vi "Test Initiate.vi"(0 "Template Rx Test in":refnum<class "niDTS WLAN Rx Test.lvclass">, 11 "error in (no error)":errorcluster) -> (4 "Template Rx Test out":refnum<class "niDTS WLAN Rx Test.lvclass">, 15 "error out":errorcluster)   [LabVIEW 2015, in "niDTS WLAN.lvlib" / "niDTS WLAN Rx Test.lvclass"]
uses:
  niDTS WLAN Rx Test.lvclass
  niDTS WLAN Rx Test.lvclass/niDTS WLAN Rx Test.ctl
  Instrument/INSTR RX/niDTS WLAN INSTR RX.lvclass
  Framework/Dut/Objects/BASE_class/niDTS Dut.lvclass
  Dut/Objects/BASE_class/niDTS WLAN Dut.lvclass
  niDTS WLAN.lvlib
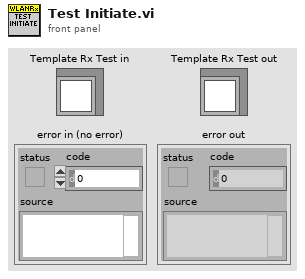
[diagram p1: front panel]
types:
  T1 = typedef "niDTS Framework.lvlib/niDTS Dut INC Handle.ctl" = refnum<data-value>
  T2 = typedef "niDTS WLAN.lvlib/niDTS WLAN Dut INC Handle.ctl" = refnum<data-value>
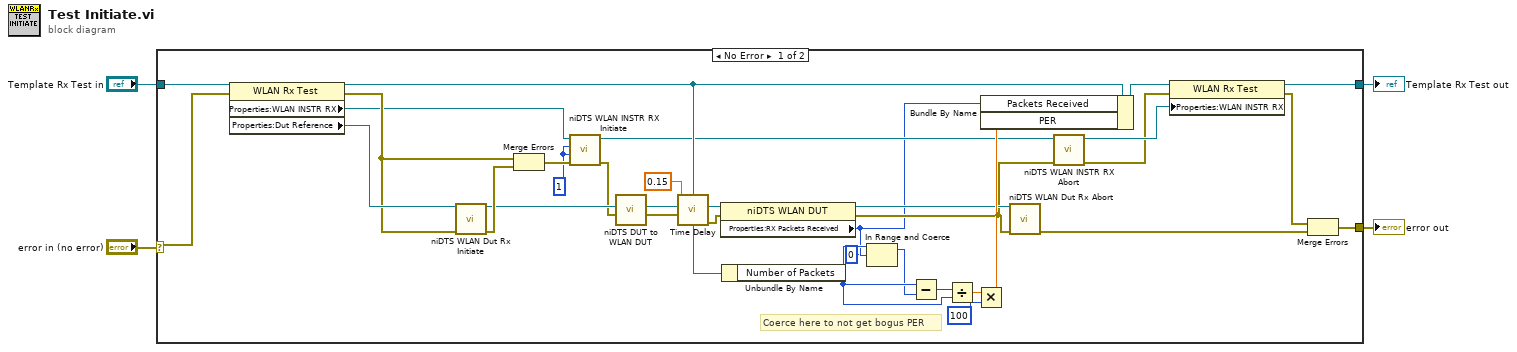
[diagram p0: block diagram]
diagram:
  n1 = case shown="No Error" "error in (no error)" {
    selector: "error in (no error)" -> [w37 w39]
    tunnel: [w12 w39] -> w3
    tunnel: [w11 w38] -> w1
    tunnel: "Template Rx Test in" -> [w36 w38]
    frame No Error {
      w27 = 1 ("Driver Instance")
      # "Coerce here to not get bogus PER"
      n2 = property class="WLAN Rx Test"(reference=w36, error in=w37) -> (reference out=w29:refnum<class "niDTS WLAN Rx Test.lvclass">, error out=w26:errorcluster, "Properties:WLAN INSTR RX"=w19:refnum<class "niDTS WLAN INSTR RX.lvclass">, "Properties:Dut Reference"=w35:T1)
      n3 = call "niDTS WLAN Dut Rx Initiate.vi"("Dut Handle in"=w35, "error in (no error)"=w26) -> ("Dut Handle out"=w23:T1, "error out"=w25:errorcluster)  [unwired: 12 in]
      n4 = Merge Errors(w26, w25) -> (w28:errorcluster)
      n5 = call-dynamic "niDTS WLAN INSTR RX Initiate.vi"("error in (no error)"=w28, "Result Instance"=w27, "Driver Instance"=w27, "niDTS WLAN INSTR RX in"=w19) -> ("error out"=w22:errorcluster, "niDTS WLAN INSTR RX out"=w20:refnum<class "niDTS WLAN INSTR RX.lvclass">)  [unwired: 6 in]
      n6 = call "niDTS DUT to WLAN DUT.vi"("error in"=w22, "Dut Handle"=w23) -> ("error out"=w18:errorcluster, "WLAN Dut Handle"=w21:T2)  [unwired: 8 in]
      n7 = call "Time Delay"("error in (no error)"=w18, "Delay Time (s)"=0.15) -> ("error out"=w17:errorcluster)  [unwired: 9 in]
      n8 = property class="niDTS WLAN DUT"(reference=w21, error in=w17) -> (reference out=w30:T2, error out=w9:errorcluster, "Properties:RX Packets Received"=w7:u32)
      n9 = Unbundle By Name(w29) -> ("Number of Packets"=w8:i32)
      n10 = In Range and Coerce(upper limit=w8, x=w7, lower limit=u32 0) -> (coerced(x)=w5:u32)  [unwired: 1 out]
      n11 = Subtract(x=w8, y=w5) -> (x-y=w34:u32)
      n12 = Divide(x=w34, y=w8) -> (x/y=w33:dbl)
      n13 = Multiply(x=w33, y=100 ("Parameters.RX Measurement Parameters.Number of Packets")) -> (x*y=w31:dbl)
      n14 = Bundle By Name(cluster=w29, "Packets Received"=w7, "PER"=w31) -> (w16:refnum<class "niDTS WLAN Rx Test.lvclass">)
      n15 = call "niDTS WLAN Dut Rx Abort.vi"("WLAN Dut Handle in"=w30, "error in (no error)"=w9) -> ("error out"=w10:errorcluster)  [unwired: 12 in, 1 out]
      n16 = call-dynamic "niDTS WLAN INSTR RX Abort.vi"("error in (no error)"=w9, "niDTS WLAN INSTR RX in"=w20) -> ("error out"=w14:errorcluster, "niDTS WLAN INSTR RX out"=w15:refnum<class "niDTS WLAN INSTR RX.lvclass">)  [unwired: 8 in]
      n17 = property class="WLAN Rx Test"(reference=w16, error in=w14, "Properties:WLAN INSTR RX"=w15) -> (reference out=w11:refnum<class "niDTS WLAN Rx Test.lvclass">, error out=w13:errorcluster)
      n18 = Merge Errors(w13, w10) -> (w12:errorcluster)
    }
    frame Error {
    }
  }
  "error out" <- w3
  "Template Rx Test out" <- w1
